vi "read_controllo.vi"(0 "Radio Buttons":enum32{"Radio Selection 1", "Radio Selection 2"}(radio), 1 "Radio Buttons 5":enum32{"Radio Selection 1", "Radio Selection 2"}(radio), 2 "Radio Buttons 2":enum32{"Radio Selection 1", "Radio Selection 2"}(radio), 3 "Radio Buttons 3":enum32{"Radio Selection 1", "Radio Selection 2"}(radio), 4 "Radio Buttons 6":enum32{"Radio Selection 1", "Radio Selection 2"}(radio), 5 "Radio Buttons 4":enum32{"Radio Selection 1", "Radio Selection 2"}(radio), 6 "Radio Buttons 7":enum32{"Radio Selection 1", "Radio Selection 2"}(radio), 7 "Radio Buttons 8":enum32{"Radio Selection 1", "Radio Selection 2"}(radio)) -> (8 "output cluster":T1)   [LabVIEW 2019]
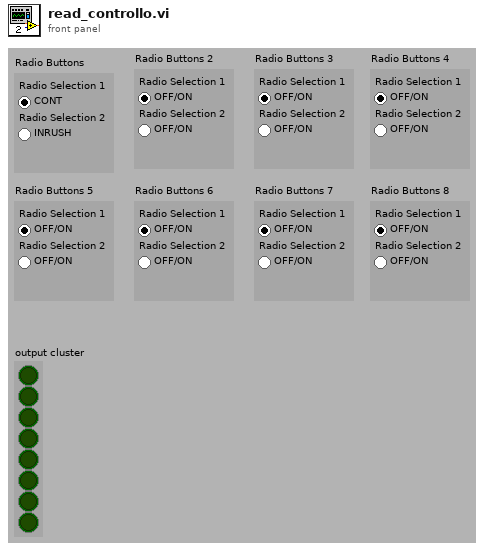
[diagram p1: front panel]
types:
  T1 = cluster{bool, bool, bool, bool, bool, bool, bool, bool}
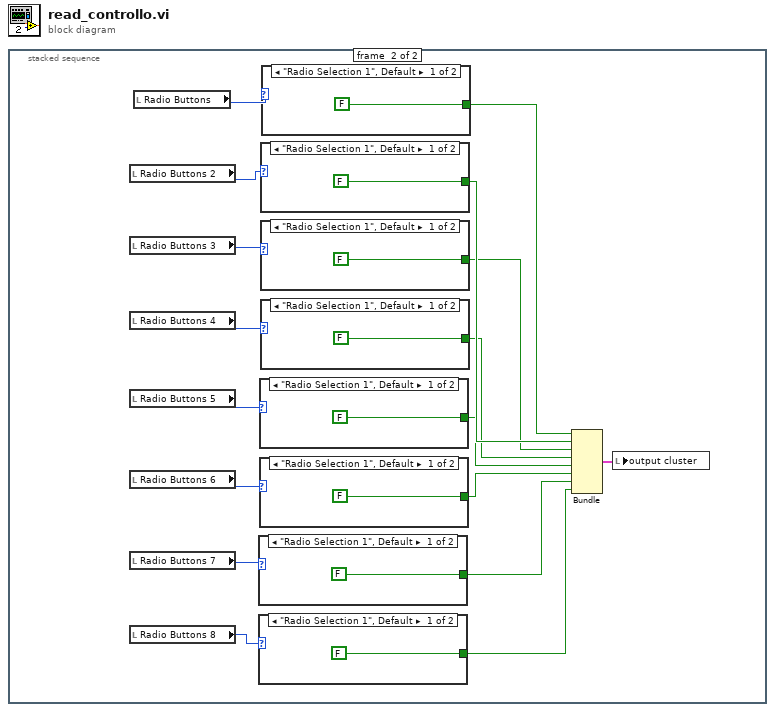
[diagram p0: block diagram]
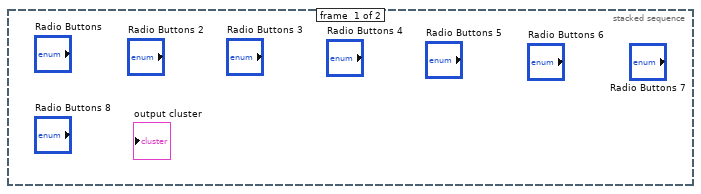
[diagram p2: hidden frame]
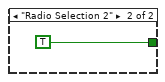
[diagram p3: hidden frame]
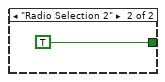
[diagram p4: hidden frame]
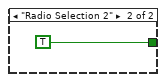
[diagram p5: hidden frame]
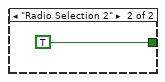
[diagram p6: hidden frame]
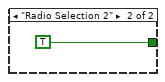
[diagram p7: hidden frame]
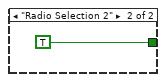
[diagram p8: hidden frame]
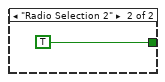
[diagram p9: hidden frame]
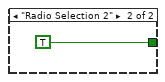
[diagram p10: hidden frame]
diagram:
  n1 = stacked-sequence {
    frame #0 {
    }
    frame #1 {
      n2 = local read "Radio Buttons 2"() -> (w8:enum32{"Radio Selection 1", "Radio Selection 2"})
      n3 = local read "Radio Buttons 3"() -> (w7:enum32{"Radio Selection 1", "Radio Selection 2"})
      n4 = local read "Radio Buttons 4"() -> (w6:enum32{"Radio Selection 1", "Radio Selection 2"})
      n5 = local read "Radio Buttons 5"() -> (w5:enum32{"Radio Selection 1", "Radio Selection 2"})
      n6 = local read "Radio Buttons 6"() -> (w4:enum32{"Radio Selection 1", "Radio Selection 2"})
      n7 = local read "Radio Buttons 7"() -> (w3:enum32{"Radio Selection 1", "Radio Selection 2"})
      n8 = local read "Radio Buttons 8"() -> (w2:enum32{"Radio Selection 1", "Radio Selection 2"})
      n9 = local read "Radio Buttons"() -> (w9:enum32{"Radio Selection 1", "Radio Selection 2"})
      n10 = case shown="\"Radio Selection 1\", Default" w3 {
        tunnel: [FALSE TRUE] -> w11
        frame "Radio Selection 1", Default {
        }
        frame "Radio Selection 2" {
        }
      }
      n11 = case shown="\"Radio Selection 1\", Default" w2 {
        tunnel: [FALSE TRUE] -> w10
        frame "Radio Selection 1", Default {
        }
        frame "Radio Selection 2" {
        }
      }
      n12 = case shown="\"Radio Selection 1\", Default" w5 {
        tunnel: [FALSE TRUE] -> w13
        frame "Radio Selection 1", Default {
        }
        frame "Radio Selection 2" {
        }
      }
      n13 = case shown="\"Radio Selection 1\", Default" w4 {
        tunnel: [FALSE TRUE] -> w12
        frame "Radio Selection 1", Default {
        }
        frame "Radio Selection 2" {
        }
      }
      n14 = case shown="\"Radio Selection 1\", Default" w8 {
        tunnel: [FALSE TRUE] -> w16
        frame "Radio Selection 1", Default {
        }
        frame "Radio Selection 2" {
        }
      }
      n15 = case shown="\"Radio Selection 1\", Default" w7 {
        tunnel: [FALSE TRUE] -> w15
        frame "Radio Selection 1", Default {
        }
        frame "Radio Selection 2" {
        }
      }
      n16 = case shown="\"Radio Selection 1\", Default" w6 {
        tunnel: [FALSE TRUE] -> w14
        frame "Radio Selection 1", Default {
        }
        frame "Radio Selection 2" {
        }
      }
      n17 = case shown="\"Radio Selection 1\", Default" w9 {
        tunnel: [FALSE TRUE] -> w17
        frame "Radio Selection 1", Default {
        }
        frame "Radio Selection 2" {
        }
      }
      n18 = Bundle(w17, w16, w15, w14, w13, w12, w11, w10) -> (w1:T1)  [unwired: 1 in]
      n19 = local write "output cluster"(w1) -> ()
    }
  }
